vi "ActionVIOnCompile.vi"(8 "error in (no error)":errorcluster, 11 "Device Item Ref in":T1 format="%.0x") -> (0 "error out":errorcluster)   [LabVIEW 2016, in "FPGA Addon System Explorer.lvlib"]
uses:
  FPGA Addon System Explorer.lvlib
  <vilib>/NI Veristand/Custom Device API/Custom Device Item Ref.ctl
  <vilib>/NI Veristand/Custom Device API/Data Access Type.ctl
  FPGA-Resource-Manager-APIs/Source/Shared/FG Action.ctl
  Shared/Compiled.Settings.ctl
  Shared/Compiled.RegisterSettings.ctl
  Shared/Scalar Type.ctl
  Shared/Register Information.ctl
  FPGA-Resource-Manager-APIs/Source/Shared/Data Type.ctl
  <vilib>/NI Veristand/Custom Device API/Block Data Reference.ctl
  <vilib>/NI Veristand/Custom Device API/Data Reference.ctl
  Shared/Compiled.DMASettings.ctl
  Shared/DMA Settings.ctl
  Shared/Delacing Scheme.ctl
  Shared/DMA Acquisition Mode.ctl
  <vilib>/NI Veristand/Custom Device API/Waveform Data Reference.ctl
  FPGA-Resource-Manager-APIs/Source/Shared/FPGA Settings.ctl
  <vilib>/NI Veristand/Custom Device API/Custom Device Target Type.ctl
  Shared/Available Registers FG.vi
  FPGA-Resource-Manager-APIs/Source/System Definition/API/Server-Specific/Resource Groups/get fpga resources compatible with FPGA Addon CD group.vi
  Shared/Constants.vi
  <vilib>/NI Veristand/Custom Device API/NI VeriStand - Get Item Property.vi
  <vilib>/NI Veristand/Custom Device API/Get Item Property (Path).vi
  <vilib>/NI Veristand/Custom Device API/Get Item Property (String).vi
  <vilib>/NI Veristand/Custom Device API/Set Item Property (Path).vi
  <vilib>/NI Veristand/Custom Device API/Set Item Property (String).vi
  <vilib>/NI Veristand/Custom Device Tools/Custom Device Utility Library/NI VeriStand - Search for Item.vi
  <vilib>/NI Veristand/Custom Device Tools/Custom Device Utility Library/NI VeriStand - Search for Item by GUID.vi
  FPGA-Resource-Manager-APIs/Source/Shared/find Relative VS Ref.vi
  FPGA-Resource-Manager-APIs/Source/System Definition/API/FPGA Resource Discovery/get FPGA resources for this FPGA Addon CD.vi
  SubVIs/RegMap to Register Information.vi
  <vilib>/NI Veristand/Custom Device API/NI VeriStand - Get Item Children.vi
  <vilib>/NI Veristand/Custom Device API/NI VeriStand - Get Custom Device Channel Data.vi
  <vilib>/NI Veristand/Custom Device API/Set Item Property (Variant).vi
  <vilib>/NI VeriStand/Custom Device API/Custom Device API.lvlib
  Shared/FPGA Addon Shared.lvlib
  FPGA-Resource-Manager-APIs/Source/Shared/FPGA RM Shared API.lvlib
  <vilib>/NI/NIVS Inline Async API/_Data Access System Explorer/Data Access System Explorer.lvlib
  <vilib>/NI VeriStand/Custom Device Tools/Custom Device Utility Library/Custom Device Utility Library.lvlib
  FPGA-Resource-Manager-APIs/Source/System Definition/FPGA RM System Definition API.lvlib
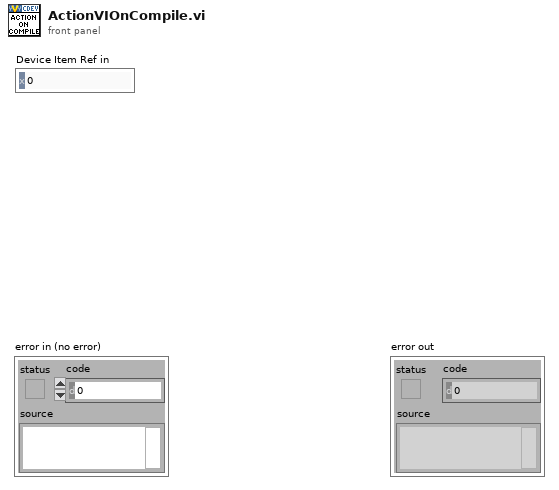
[diagram p1: front panel]
types:
  T1 = typedef "Custom Device API.lvlib/Custom Device Item Ref.ctl" = u64
  T2 = typedef "FPGA Addon Shared.lvlib/Compiled.Settings.ctl" = cluster{"Name":string, "IncomingRegisters.Settings":T3[], "IncomingRegisters.Refs":cluster{"Refs":T7[], "Values":dbl[]}, "OutgoingRegisters.Settings":T3[], "OutgoingRegisters.Refs":cluster{"Refs":T7[], "Values":dbl[]}, "Incoming.Size":i32, "Outgoing.Size":i32, "IncomingDMA.Settings":T9[], "OutgoingDMA.Settings":T9[], "FPGA.Settings":T14, "Target.Type":T15}
  T3 = typedef "FPGA Addon Shared.lvlib/Compiled.RegisterSettings.ctl" = cluster{"Scalar Type":T4, "Index":i32, "Length":i32, "Register":T5}
  T4 = typedef "FPGA Addon Shared.lvlib/Scalar Type.ctl" = enum16{"Standard", "Bitpacked"}
  T5 = typedef "FPGA Addon Shared.lvlib/Register Information.ctl" = cluster{"Name":string, "Data Type":T6, "Default Value":variant}
  T6 = typedef "FPGA RM Shared API.lvlib/Data Type.ctl" = enum8{"<Null>", "I8", "I16", "I32", "I64", "U8", "U16", "U32", "U64", "SGL", "Boolean", "Analog PWM In Settings", "Analog PWM In", "Digital PWM In Settings", "Digital PWM In", "Digital PWM Out", "Sine Out", "FXP+/-24.5", "FXP+/-16.5", "FXP+/-32.8", "FXP+/-64.32", "FXP+/-16.7", "FXP+/-20.5"}
  T7 = typedef "Custom Device API.lvlib/Block Data Reference.ctl" = cluster{"Data Reference":T8, "Offset":u64, "Length":u64}
  T8 = typedef "Custom Device API.lvlib/Data Reference.ctl" = i32
  T9 = typedef "FPGA Addon Shared.lvlib/Compiled.DMASettings.ctl" = cluster{"Name":string, "DMA.Settings":T10, "DMA.VSRefs":T13[]}
  T10 = typedef "FPGA Addon Shared.lvlib/DMA Settings.ctl" = cluster{"Number of Channels":u8, "Delacing Scheme":T11, "Update Rate":u32, "dt":dbl, "Mode":T12, "Number of Samples":u32, "DMA Host Buffer":u32}
  T11 = typedef "FPGA Addon Shared.lvlib/Delacing Scheme.ctl" = enum8{"Interleaved"}
  T12 = typedef "FPGA Addon Shared.lvlib/DMA Acquisition Mode.ctl" = enum8{"Continuous", "Triggered Finite"}
  T13 = typedef "Custom Device API.lvlib/Waveform Data Reference.ctl" = i32
  T14 = typedef "FPGA RM Shared API.lvlib/FPGA Settings.ctl" = cluster{"Bitfile path":path, "RIO Device Address":string}
  T15 = typedef "Custom Device API.lvlib/Custom Device Target Type.ctl" = enum16{"PharLap", "VxWorks", "Windows", "Linux_32_ARM", "Linux_x64"}
  T16 = typedef "Custom Device API.lvlib/Data Access Type.ctl" = enum16{"Read", "Write"}
  T17 = typedef "FPGA RM Shared API.lvlib/FG Action.ctl" = enum8{"GET", "SET"}
  T18 = typedef "Custom Device API.lvlib/Custom Device Item Info.ctl" = cluster{"Name":string, "Is Channel":bool, "GUID":string, "Is Waveform":bool}
  T19 = cluster{"Name":string, "Type":enum16{"Output/Write", "Input/Read", "Input/ReadWrite"}, "VS Refs":T1[]}[]
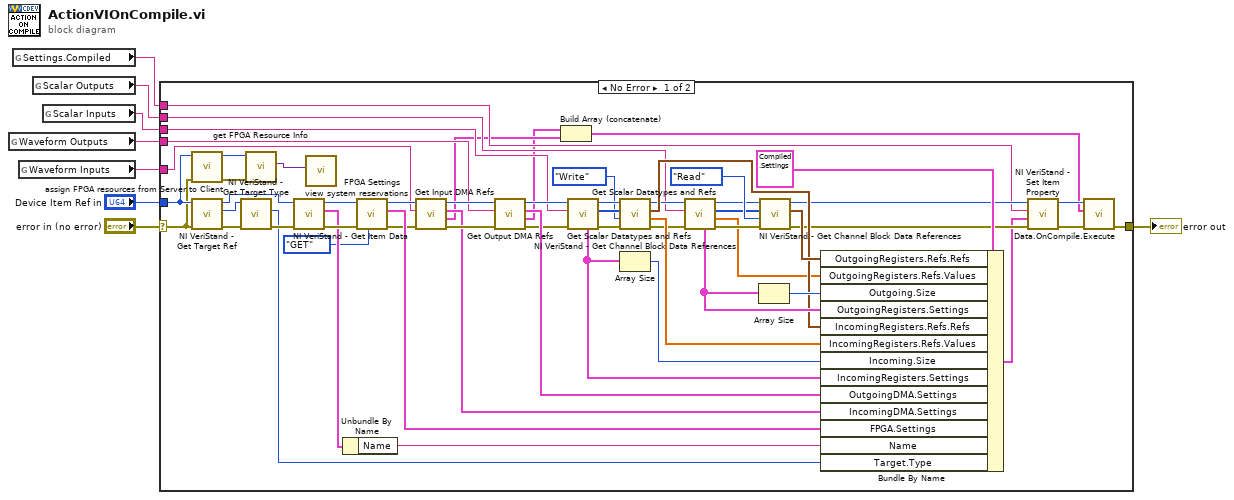
[diagram p0: block diagram]
diagram:
  n1 = global read "Constants.vi" "Waveform Outputs"() -> (w4:string)
  n2 = global read "Constants.vi" "Settings.Compiled"() -> (w1:string)
  n3 = global read "Constants.vi" "Waveform Inputs"() -> (w5:string)
  n4 = global read "Constants.vi" "Scalar Outputs"() -> (w2:string)
  n5 = global read "Constants.vi" "Scalar Inputs"() -> (w3:string)
  n6 = case shown="No Error" "error in (no error)" {
    selector: "error in (no error)" -> [w12 w66]
    tunnel: [w22 w66] -> w7
    tunnel: "Device Item Ref in" -> [w13 _]
    tunnel: w5 -> [w32 _]
    tunnel: w4 -> [w31 _]
    tunnel: w3 -> [w30 _]
    tunnel: w2 -> [w29 _]
    tunnel: w1 -> [w26 _]
    frame No Error {
      n7 = call "assign FPGA resources from Server to Client.vi"("error in (no error)"=w12, "Device Item Ref in"=w13) -> ("error out"=w11:errorcluster, "Device Item Ref out"=w10:T1)  [unwired: 8 in]
      n8 = call <vilib>:"NI VeriStand - Get Target Ref.vi"("error in"=w12, "Item Ref in"=w13) -> ("error out"=w19:errorcluster, "Target Ref"=w18:T1, "Item Ref out"=w16:T1)  [unwired: 6 in, 1 out]
      n9 = call <vilib>:"NI VeriStand - Get Target Type.vi"("error in (no error)"=w19, "Item Ref in"=w18) -> ("error out"=w17:errorcluster, "Target Type"=w15:T15)  [unwired: 7 in, 1 out]
      n10 = call "get FPGA Resource Info.vi"("error in (no error)"=w11, "CD Ref in"=w10) -> ("Value"=w9:variant)  [unwired: 7 in, 2 out]
      n11 = call <vilib>:"NI VeriStand - Get Item Data.vi"("error in (no error)"=w17, "Item Ref in"=w16) -> ("error out"=w63:errorcluster, "Item Info"=w51:T18, "Item Ref out"=w62:T1)  [unwired: 6 in, 1 out]
      n12 = call "view system reservations.vi"("Variant"=w9) -> ()  [unwired: 11 in]
      n13 = Unbundle By Name(w51) -> ("Name"=w52:string)
      n14 = call "FPGA Settings.vi"("Action"=FG_Action."GET", "error in (no error)"=w63, "Item Ref"=w62) -> ("error out"=w64:errorcluster, "FPGA Settings"=w65:T14, "Item Ref out"=w53:T1)  [unwired: 6 in]
      n15 = call "Get Input DMA Refs.vi"("error in (no error)"=w64, "Item GUID"=w32, "Section Ref in"=w53) -> ("error out"=w55:errorcluster, "Refs"=w25:T19, "DMA Settings"=w54:T9[], "Section Ref out"=w57:T1)  [unwired: 5 in]
      n16 = call "Get Output DMA Refs.vi"("error in (no error)"=w55, "Item GUID"=w31, "Section Ref in"=w57) -> ("error out"=w56:errorcluster, "Refs"=w24:T19, "DMA"=w59:T9[], "Section Ref out"=w58:T1)  [unwired: 5 in]
      n17 = Build Array (concatenate)(w24, w25) -> (w20:T19)
      n18 = call "Get Scalar Datatypes and Refs.vi"("error in (no error)"=w56, "Item GUID"=w30, "Section Ref in"=w58) -> ("error out"=w37:errorcluster, "VS Ref"=w35:T1[], "Section Ref out"=w36:T1, "Registers Ref"=w60:T3[])  [unwired: 4 in, 1 out]
      n19 = call <vilib>:"NI VeriStand - Get Channel Block Data References.vi"("error in (no error)"=w37, "Access"=Data_Access_Type."Write", "Channel Refs"=w35, "Device Ref in"=w36) -> ("error out"=w38:errorcluster, "Values Array"=w50:dbl[], "Block Data Refs"=w46:T7[], "Device Ref out"=w39:T1)  [unwired: 4 in]
      n20 = Array Size(array=w60) -> (size(s)=w49:i32)
      n21 = call "Get Scalar Datatypes and Refs.vi"("error in (no error)"=w38, "Item GUID"=w29, "Section Ref in"=w39) -> ("error out"=w41:errorcluster, "Default Values"=w14:dbl[], "VS Ref"=w43:T1[], "Section Ref out"=w42:T1, "Registers Ref"=w61:T3[])  [unwired: 4 in]
      n22 = Array Size(array=w61) -> (size(s)=w48:i32)
      n23 = call <vilib>:"NI VeriStand - Get Channel Block Data References.vi"("error in (no error)"=w41, "Access"=Data_Access_Type."Read", "Channel Refs"=w43, "Device Ref in"=w42) -> ("error out"=w33:errorcluster, "Block Data Refs"=w47:T7[], "Device Ref out"=w27:T1)  [unwired: 4 in, 1 out]
      n24 = Bundle By Name(cluster=T2 {"Name"="", "IncomingRegisters.Settings"=[], "IncomingRegisters.Refs"={"Refs"=[], "Values"=[]}, "OutgoingRegisters.Settings"=[], "OutgoingRegisters.Refs"={"Refs"=[], "Values"=[]}, "Incoming.Size"=0, "Outgoing.Size"=0, "IncomingDMA.Settings"=[], "OutgoingDMA.Settings"=[], "FPGA.Settings"={"Bitfile path"=path "", "RIO Device Address"=""}, "Target.Type"=enum."PharLap"}, "OutgoingRegisters.Refs.Refs"=w47, "OutgoingRegisters.Refs.Values"=w14, "Outgoing.Size"=w48, "OutgoingRegisters.Settings"=w61, "IncomingRegisters.Refs.Refs"=w46, "IncomingRegisters.Refs.Values"=w50, "Incoming.Size"=w49, "IncomingRegisters.Settings"=w60, "OutgoingDMA.Settings"=w59, "IncomingDMA.Settings"=w54, "FPGA.Settings"=w65, "Name"=w52, "Target.Type"=w15) -> (w28:T2)
      n25 = call-poly <vilib>:"NI VeriStand - Set Item Property.vi"("error in (no error)"=w33, "Value"=w28, "Property Name"=w26, "Item Ref in"=w27) -> ("error out"=w23:errorcluster, "Item Ref out"=w21:T1)  [unwired: 5 in, 1 out]
      n26 = call <vilib>:"Data.OnCompile.Execute.vi"("error in"=w23, "VS Ref Groups"=w20, "Custom Device Ref"=w21) -> ("error out"=w22:errorcluster)  [unwired: 7 in, 1 out]
    }
    frame Error {
    }
  }
  "error out" <- w7
